vi "Image Preperation 3D.vi"(9 "Color Array":T1[](array[typedef]), 10 "Coordinates":T2(array[cluster])) -> (0 "Indicies":u32[](array[numeric]), 1 "Colour":T1[](array[typedef]), 2 "XYZ":cluster{"X":dbl, "Y":dbl, "Z":dbl}[](array[cluster]))   [LabVIEW 2017]
uses:
  <vilib>/Utility/miscctls.llb/LVRGBAColorTypeDef.ctl
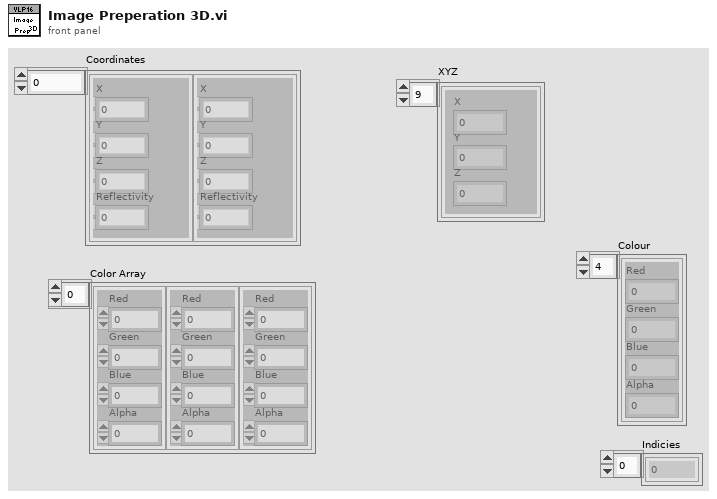
[diagram p1: front panel]
types:
  T1 = typedef "LVRGBAColorTypeDef.ctl" = cluster{"Red":sgl, "Green":sgl, "Blue":sgl, "Alpha":sgl}
  T2 = cluster{"X":dbl, "Y":dbl, "Z":dbl, "Reflectivity":dbl}[]
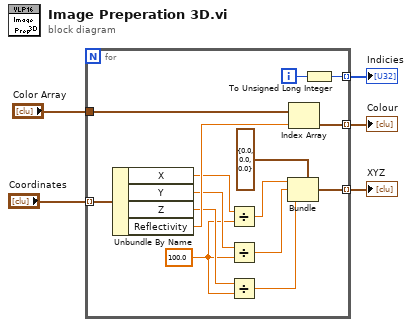
[diagram p0: block diagram]
diagram:
  n1 = for {
    tunnel: "Coordinates" -> [w20] mode=indexing
    tunnel: "Color Array" -> [w19]
    tunnel: [w18] -> w3 mode=indexing
    tunnel: [w16] -> w2 mode=indexing
    tunnel: [w14] -> w1 mode=indexing
    i -> [w17]
    w9 = 100.0 ("y")
    n2 = Unbundle By Name(w20) -> ("X"=w12:dbl, "Y"=w11:dbl, "Z"=w10:dbl, "Reflectivity"=w13:dbl)
    n3 = Divide(x=w12, y=w9) -> (x/y=w8:dbl)
    n4 = Divide(x=w11, y=w9) -> (x/y=w7:dbl)
    n5 = Divide(x=w10, y=w9) -> (x/y=w6:dbl)
    n6 = Bundle(cluster=cluster{"X":dbl, "Y":dbl, "Z":dbl} {"X"=0.0, "Y"=0.0, "Z"=0.0}, "X"=w8, "Y"=w7, "Z"=w6) -> (w14:cluster{"X":dbl, "Y":dbl, "Z":dbl})
    n7 = Index Array(array=w19, index=w13) -> (element=w18:T1)
    n8 = To Unsigned Long Integer(number=w17) -> (unsigned 32bit integer=w16:u32)
  }
  "XYZ" <- w1
  "Colour" <- w3
  "Indicies" <- w2
